vi "CODCr水质测量数据table定义.vi"(5 "数据类型":enum16{"N", "M"}(ring)=enum."M", 7 "table 输入":string, 9 "SN":string, 10 "测量模式":T1(ring)=enum."水样测试", 11 "data":T3 {"单位" items=["ug/L", "mg/L", "ppm", "mg/m3", "cm", "ppb", "ug/m3", "%", "nmol/mol", "umol/mol", "MPN/L", "MPN/100ml", "ng/m3", "NTU", "无量纲", "ms/cm", "us/cm"]}) -> (1 "table 输出":string, 2 "columns":string[](array[string]), 3 "data输出":T2)   [LabVIEW 2016, in "CODCr库.lvlib"]
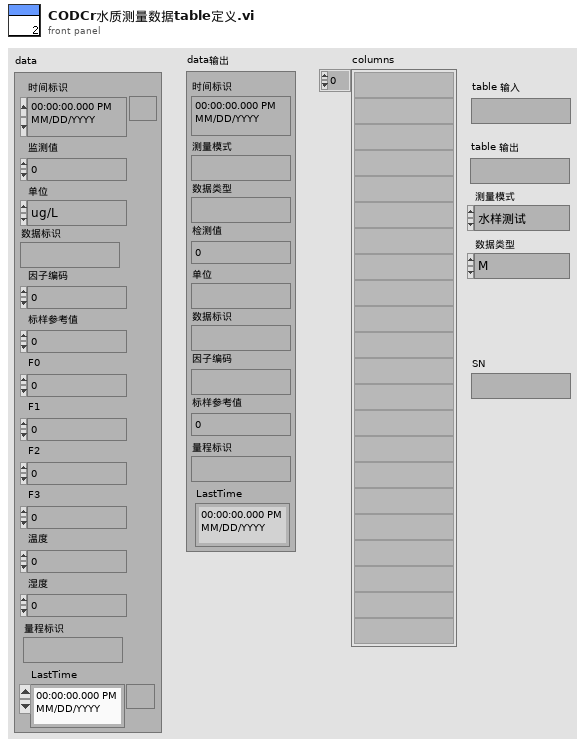
[diagram p1: front panel]
types:
  T1 = enum16{"空闲", "水样测试", "标样核查", "零点核查", "跨度核查", "空白测试", "平行样测试", "加标回收", "空白校准", "标样校准", "初始化（清洗）"}
  T2 = cluster{"时间标识":timestamp, "测量模式":string, "数据类型":string, "检测值":sgl, "单位":string, "数据标识":string, "因子编码":string, "标样参考值":sgl, "量程标识":string, "LastTime":timestamp}
  T3 = cluster{"时间标识":timestamp, "监测值":sgl, "单位":u16, "数据标识":string, "因子编码":u32, "标样参考值":sgl, "F0":sgl, "F1":sgl, "F2":sgl, "F3":sgl, "温度":sgl, "湿度":sgl, "量程标识":string, "LastTime":timestamp}
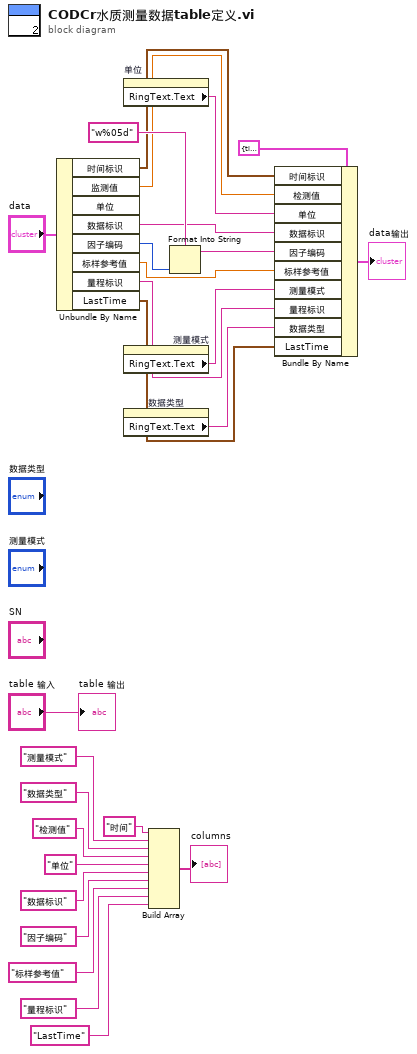
[diagram p0: block diagram]
diagram:
  n1 = Unbundle By Name("data") -> ("时间标识"=w17:timestamp, "监测值"=w16:sgl, "数据标识"=w15:string, "因子编码"=w21:u32, "标样参考值"=w12:sgl, "量程标识"=w7:string, "LastTime"=w3:timestamp)  [unwired: 1 out]
  n2 = property on="单位" class="Ring (严格)"() -> ("RingText.Text"=w14:string)  [unwired: 2 in, 2 out]
  n3 = property on="测量模式" class="Enum (严格)"() -> ("RingText.Text"=w8:string)  [unwired: 2 in, 2 out]
  n4 = property on="数据类型" class="Enum (严格)"() -> ("RingText.Text"=w6:string)  [unwired: 2 in, 2 out]
  n5 = Build Array("时间", "测量模式", "数据类型", "检测值", "单位", "数据标识", "因子编码", "标样参考值", "量程标识", "LastTime" ("元素")) -> (→"columns":string[])
  n6 = Format Into String(format string="w%05d" ("格式字符串"), w21) -> (resulting string=w18:string)  [unwired: 2 in, 1 out]
  n7 = Bundle By Name(cluster=T2 {"时间标识"=timestamp(0 s since 1904-01-01), "测量模式"="", "数据类型"="", "检测值"=0.0, "单位"="", "数据标识"="", "因子编码"="", "标样参考值"=0.0, "量程标识"="", "LastTime"=timestamp(0 s since 1904-01-01)} ("data输出"), "时间标识"=w17, "检测值"=w16, "单位"=w14, "数据标识"=w15, "因子编码"=w18, "标样参考值"=w12, "测量模式"=w8, "量程标识"=w7, "数据类型"=w6, "LastTime"=w3) -> (→"data输出":T2)
  "table 输出" <- "table 输入"
